vi "Video Window Handler_ABB.vi"(9 "Action":T1=enum."Hide", 10 "This VI":refnum<vi>, 11 "Video Displays":T2) -> ()   [LabVIEW 2017]
uses:
  <vilib>/Utility/miscctls.llb/LVBoundsTypeDef.ctl
  <vilib>/Utility/miscctls.llb/LVPointTypeDef.ctl
  Video Display Buttons.ctl
  Video Command type.ctl
  VideoWindowsCommand.ctl
  ABB global.vi
panel:
  out "Screen Coordinates":T3
  out "Bounds":T4
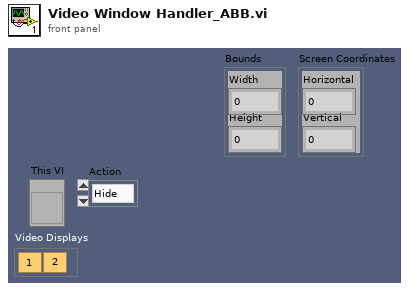
[diagram p1: front panel]
types:
  T1 = typedef "Video Command type.ctl" = enum16{"Show", "Hide", "Exit", "Kick"}
  T2 = typedef "Video Display Buttons.ctl" = cluster{"1":bool, "1 2":bool}
  T3 = typedef "LVPointTypeDef.ctl" = cluster{"Horizontal":i16, "Vertical":i16}
  T4 = typedef "LVBoundsTypeDef.ctl" = cluster{"Width":u32, "Height":u32}
  T5 = typedef "VideoWindowsCommand.ctl" = cluster{"Position":cluster{"Right":i32, "Bottom":i32}, "Action":T1, "Camera Addresses":cluster{"Camera 1":string, "Camera 2":string, "Mobile":string}}
  T6 = cluster{"Camera 1":string, "Camera 2":string, "Mobile":string}
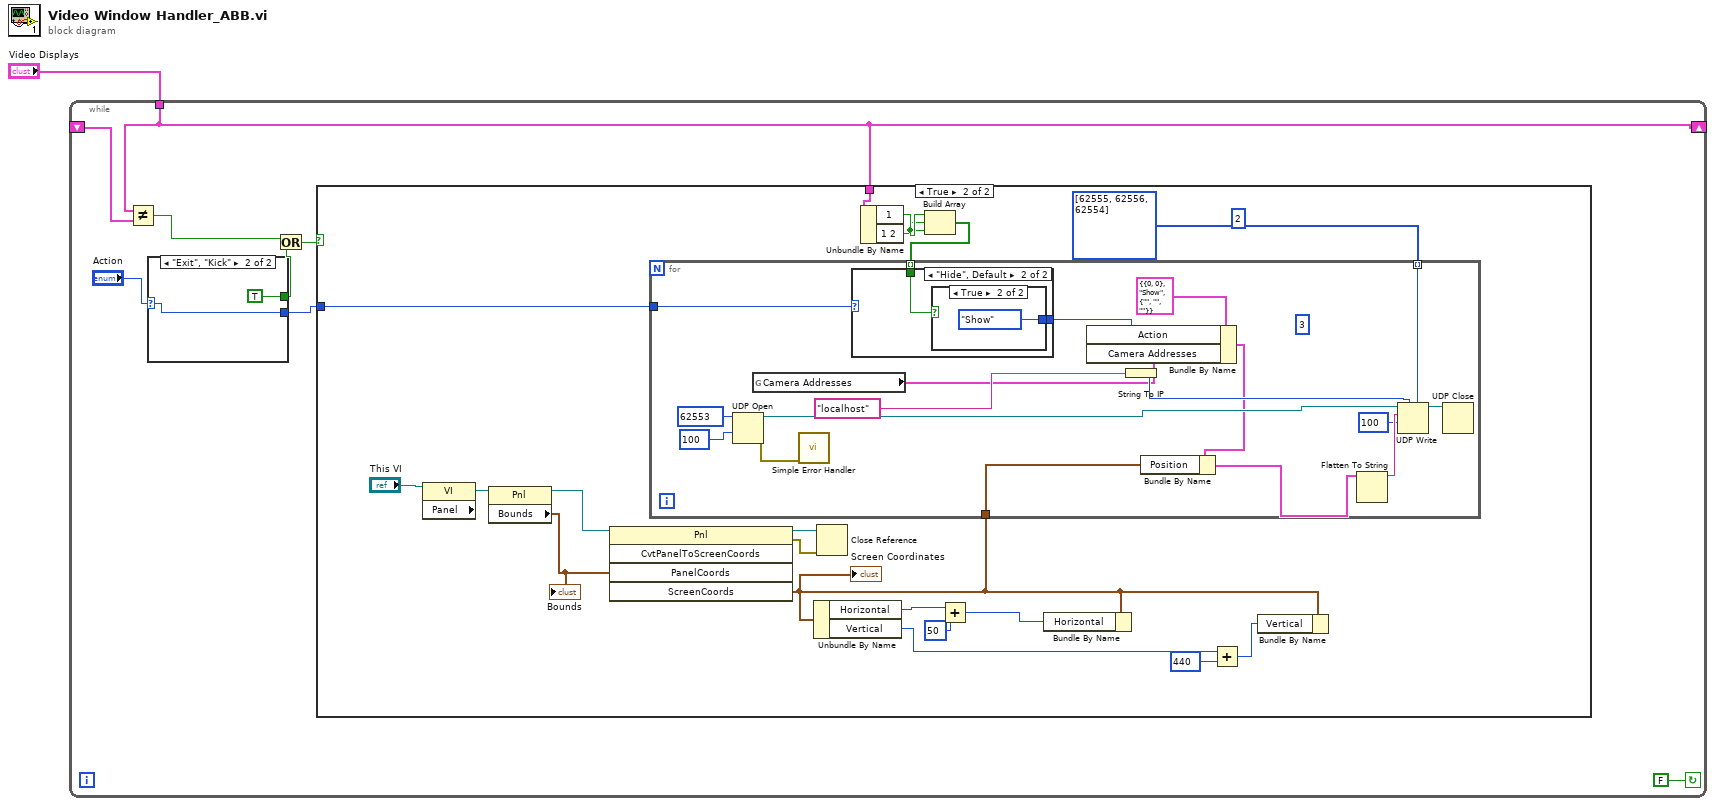
[diagram p0: block diagram]
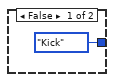
[diagram p5: hidden frame]
diagram:
  n1 = while {
    shift-right: [w7] -> _
    shift-left: _ -> [w8]
    tunnel: "Video Displays" -> [w7]
    stop <- FALSE continue-if-true
    n2 = Not Equal?(x=w7, y=w8) -> (x != y?=w6:bool)
    n3 = case shown="\"Exit\", \"Kick\"" "Action" {
      selector: "Action" -> [_ w10]
      tunnel: [_ TRUE] -> w3
      tunnel: [_ w10] -> w2
      frame "Show", Default {
      }
      frame "Exit", "Kick" {
      }
    }
    n4 = Or(x=w6, y=w3) -> (x .or. y?=w5:bool)
    n5 = case shown="True" w5 {
      tunnel: w7 -> [_ w15]
      tunnel: w2 -> [_ w16]
      frame False {
      }
      frame True {
        (unwired) 2
        n6 = property class="VI"(reference="This VI") -> ("Panel"=w28:refnum<vi>)  [unwired: 1 in, 2 out]
        n7 = property class="Pnl"(reference=w28) -> (reference out=w20:refnum<vi>, "Bounds"=w19:T4)  [unwired: 1 in, 1 out]
        "Bounds" <- w19
        n8 = invoke class="Pnl" method="CvtPanelToScreenCoords"(reference=w20, "PanelCoords"=w19) -> (reference out=w30:refnum<vi>, error out=w29:errorcluster, "ScreenCoords"=w18:T3)  [unwired: 3 in, 2 out]
        "Screen Coordinates" <- w18
        n9 = Unbundle By Name(w18) -> ("Horizontal"=w26:i16, "Vertical"=w23:i16)
        n10 = Close Reference(reference=w30, error in (no error)=w29) -> ()  [unwired: 1 out]
        n11 = Unbundle By Name(w15) -> ("1"=w14:bool, "1 2"=w13:bool)
        n12 = Build Array(w14, w13, w13) -> (w12:bool[])
        n13 = for {
          tunnel: w18 -> [w40]
          tunnel: u16[] [62555, 62556, 62554] -> [w34] mode=indexing
          tunnel: w12 -> [w33] mode=indexing
          tunnel: w16 -> [w31]
          (unwired) 3
          n14 = UDP Open(9:100 ("timeout ms (25000)"), 11:u16 62553 ("port")) -> (port=w46:refnum<k16>, 0:w39:errorcluster)  [unwired: 3 in, 1 out]
          n15 = global read "ABB global.vi" "Camera Addresses"() -> (w35:T6)
          n16 = call <vilib>:"Simple Error Handler.vi"("error in (no error)"=w39) -> ()  [unwired: 4 in, 5 out]
          n17 = case shown="\"Hide\", Default" w31 {
            selector: w31 -> [w49 _]
            tunnel: [w49 w51] -> w36
            tunnel: w33 -> [_ w50]
            frame "Exit" {
            }
            frame "Hide", Default {
              n18 = case shown="True" w50 {
                tunnel: [Video_Command_type."Kick" ("Action") Video_Command_type."Show" ("Action")] -> w51
                frame False {
                }
                frame True {
                }
              }
            }
          }
          n19 = Bundle By Name(cluster=T5 {"Position"={"Right"=0, "Bottom"=0}, "Action"=enum."Show", "Camera Addresses"={"Camera 1"="", "Camera 2"="", "Mobile"=""}} ("Cluster"), "Action"=w36, "Camera Addresses"=w35) -> (w37:T5)
          n20 = String To IP(1:"localhost" ("name")) -> (0:w41:u32)
          n21 = Bundle By Name(cluster=w37, "Position"=w40) -> (w42:T5)
          n22 = Flatten To String(anything=w42) -> (data string=w48:string)  [unwired: 3 in, 2 out]
          n23 = UDP Write(address=w41, port or service name=w34, connection ID=w46, data in=w48, 9:100 ("timeout ms (25000)")) -> (3:w32:refnum<k16>)  [unwired: 1 in, 1 out]
          n24 = UDP Close(connection ID=w32) -> ()  [unwired: 1 in, 2 out]
        }
        n25 = Add(x=w26, y=i16 50) -> (x+y=w24:i16)
        n26 = Bundle By Name(cluster=w18, "Horizontal"=w24) -> ()  [unwired: 1 out]
        n27 = Add(x=w23, y=i16 440) -> (x+y=w21:i16)
        n28 = Bundle By Name(cluster=w18, "Vertical"=w21) -> ()  [unwired: 1 out]
      }
    }
  }
